vi "Encoder Position & Velocity (FPGA).vi"(3 "Velocity Interval (uSec)":u32=1000, 5 "Position Reset":bool) -> (0 "Right Velocity (Counts/Interval)":i32, 1 "Right Acceleration (Counts/Interval)":i32, 2 "Right Position (Counts)":i32)   [LabVIEW 2009]
doc: "This is an FPGA vi for Quadrature Encoder Velocity and Acceleration Estimation using CompactRIO. It requires as inputs a Fixed Time Interval for velocity and acceleration estimation.\n\nThis application is designed to work with an R-Series expansion setup using PCI/PXI-7811R FPGA device and a CompactRIO cRIO-9411 digital input module installed in slot 1 of the expansion chassis."
uses:
  <vilib>/rvi/Arithmetic/AddSubMult/XNode/nirviSatArithmetic.xnode
  <vilib>/eio/EIONode/EIONode.xnode
  <vilib>/rvi/eio/nirviEIOImplementation/nirviEIOImplementation.xnode
  <vilib>/rvi/eio/common/nirviEmuTemplateMethod_noerrors.vi
  <vilib>/rvi/eio/common/nirviEmuClasses.ctl
panel:
  in  "Velocity Interval (uSec) 2":u32=1000
  out "Left Position (Counts)":i32
  out "Left Acceleration (Counts/Interval)":i32
  out "Left Velocity (Counts/Interval)":i32
  in  "stop":bool
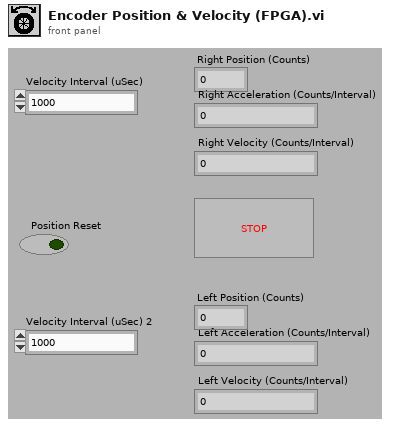
[diagram p1: front panel]
types:
  T1 = typedef "nirviEmuClasses.ctl" = enum16{"IO Read", "IO Write", "Method", "Property Read", "Property Write"}
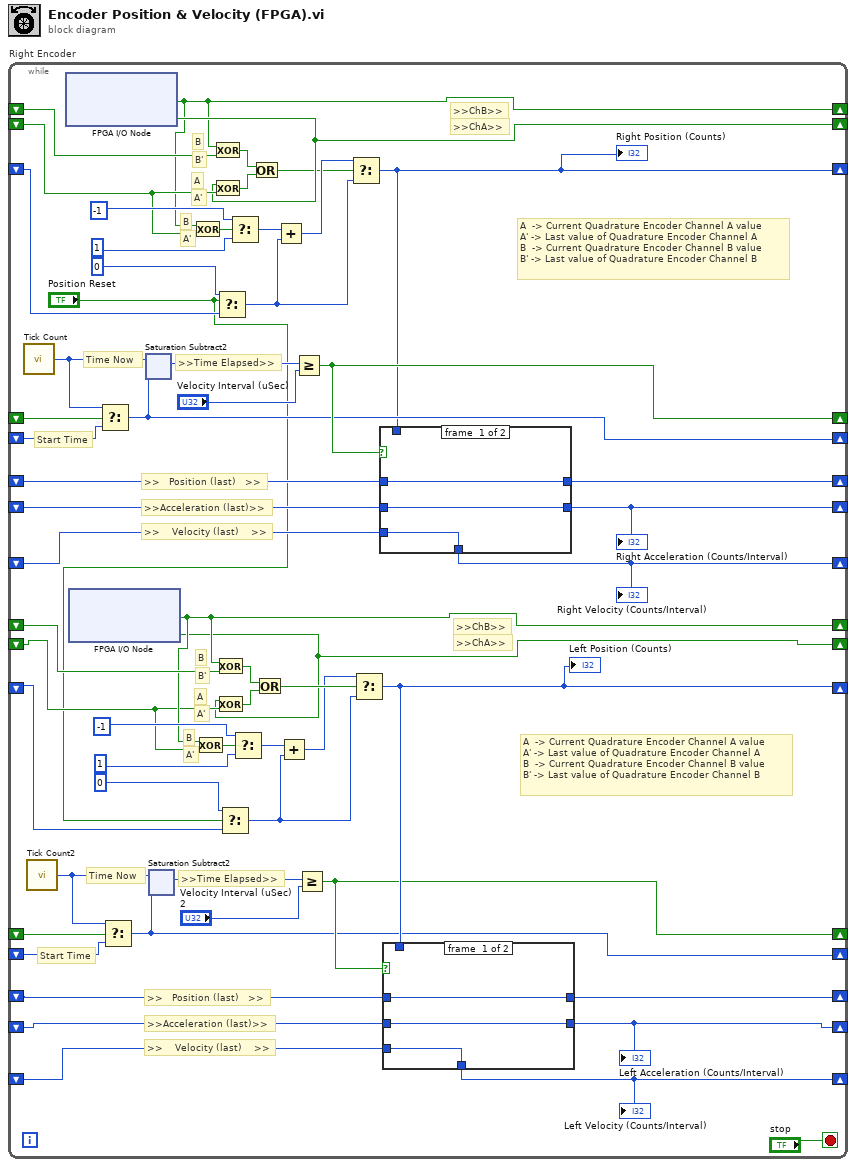
[diagram p0: block diagram]
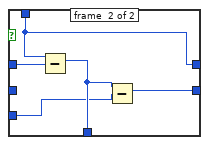
[diagram p2: hidden frame]
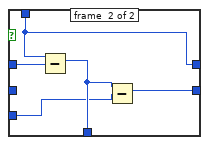
[diagram p3: hidden frame]
diagram:
  n1 = while "Right Encoder" {
    shift-right: [w32] -> _
    shift-left: _ -> [w36]
    shift-right: [w31] -> _
    shift-left: _ -> [w47]
    shift-right: [w50] -> _
    shift-left: _ -> [w51]
    shift-right: [w43] -> _
    shift-left: _ -> [w46]
    shift-right: [w38] -> _
    shift-left: _ -> [w44]
    shift-right: [w33] -> _
    shift-left: _ -> [w41]
    shift-right: [w34] -> _
    shift-left: _ -> [w40]
    shift-right: [w35] -> _
    shift-left: _ -> [w37]
    shift-right: [w16] -> _
    shift-left: _ -> [w17]
    shift-right: [w2] -> _
    shift-left: _ -> [w15]
    shift-right: [w13] -> _
    shift-left: _ -> [w14]
    shift-right: [w11] -> _
    shift-left: _ -> [w12]
    shift-right: [w9] -> _
    shift-left: _ -> [w10]
    shift-right: [w7] -> _
    shift-left: _ -> [w8]
    shift-right: [w4] -> _
    shift-left: _ -> [w6]
    shift-right: [w3] -> _
    shift-left: _ -> [w5]
    stop <- "stop" stop-if-true
    # "A  -> Current Quadrature Encoder Channel A value\nA' -> Last value of Quadrature Encoder Channel A\nB  -> Current Quadrature Encoder Channel B value\nB' -> Last value of Quadrature Encoder Channel B"
    # ">>Acceleration (last)>>"
    # "Start Time"
    # "A'"
    # "B"
    # "A'"
    # "A"
    # "B'"
    # "B"
    # ">>ChB>>"
    # ">>ChA>>"
    # ">>    Velocity (last)    >>"
    # ">>   Position (last)   >>"
    # "Time Now"
    # ">>Time Elapsed>>"
    # "A  -> Current Quadrature Encoder Channel A value\nA' -> Last value of Quadrature Encoder Channel A\nB  -> Current Quadrature Encoder Channel B value\nB' -> Last value of Quadrature Encoder Channel B"
    # ">>Acceleration (last)>>"
    # "Start Time"
    # "A'"
    # "B"
    # "A'"
    # "A"
    # "B'"
    # "B"
    # ">>ChB>>"
    # ">>ChA>>"
    # ">>    Velocity (last)    >>"
    # ">>   Position (last)   >>"
    # "Time Now"
    # ">>Time Elapsed>>"
    n2 = call "Tick Count"() -> ("Tick Count(uSec)"=w39:u32)
    n3 = call "Tick Count2"() -> ("Tick Count(uSec)"=w30:u32)
    n4 = xnode "FPGA I/O Node"() -> ("Mod2/DIO10"=w32:bool, "Mod2/DIO9"=w50:bool)  [unwired: 2 in, 2 out]
    n5 = xnode "FPGA I/O Node"() -> ("Mod2/DIO11"=w16:bool, "Mod2/DIO12"=w2:bool)  [unwired: 2 in, 2 out]
    n6 = Select(t=w39, s=w46, f=w44) -> (s? t:f=w38:u32)
    n7 = Select(t=w30, s=w12, f=w10) -> (s? t:f=w9:u32)
    n8 = xnode ("Saturation Subtract2")("x"=w39, "y"=w38) -> ("x-y"=w42:u32)
    n9 = xnode ("Saturation Subtract2")("x"=w30, "y"=w9) -> ("x-y"=w29:u32)
    n10 = Exclusive Or(1:w51, 2:w32) -> (0:w52:bool)
    n11 = Exclusive Or(1:w15, 2:w16) -> (0:w26:bool)
    n12 = Exclusive Or(1:w36, 2:w32) -> (0:w53:bool)
    n13 = Exclusive Or(1:w51, 2:w50) -> (0:w54:bool)
    n14 = Exclusive Or(1:w17, 2:w16) -> (0:w25:bool)
    n15 = Exclusive Or(1:w15, 2:w2) -> (0:w24:bool)
    n16 = Select(t=0 ("32 bit"), s="Position Reset", f=w47) -> (s? t:f=w58:i32)
    n17 = Select(t=0 ("32 bit"), s="Position Reset", f=w14) -> (s? t:f=w20:i32)
    n18 = Select(t=-1 ("32 bit"), s=w52, f=1 ("32 bit")) -> (s? t:f=w57:i32)
    n19 = Select(t=-1 ("32 bit"), s=w26, f=1 ("32 bit")) -> (s? t:f=w21:i32)
    n20 = Or(x=w53, y=w54) -> (x .or. y?=w48:bool)
    n21 = Or(x=w25, y=w24) -> (x .or. y?=w27:bool)
    n22 = Add(x=w57, y=w58) -> (x+y=w60:i32)
    n23 = Add(x=w21, y=w20) -> (x+y=w18:i32)
    n24 = Greater Or Equal?(x=w42, y="Velocity Interval (uSec)") -> (x >= y?=w43:bool)
    n25 = Greater Or Equal?(x=w29, y="Velocity Interval (uSec) 2") -> (x >= y?=w11:bool)
    n26 = Select(t=w60, s=w48, f=w58) -> (s? t:f=w31:i32)
    "Right Position (Counts)" <- w31
    n27 = Select(t=w18, s=w27, f=w20) -> (s? t:f=w13:i32)
    "Left Position (Counts)" <- w13
    n28 = case shown="True" w43 {
      tunnel: w31 -> [_ w168]
      tunnel: w41 -> [w165 w172]
      tunnel: [w167 w171] -> w34
      tunnel: w40 -> [w167 w170]
      tunnel: [w166 w169] -> w35
      tunnel: w37 -> [w166 _]
      tunnel: [w165 w168] -> w33
      frame #0 {
      }
      frame #1 {
        n29 = Subtract(x=w168, y=w172) -> (x-y=w171:i32)
        n30 = Subtract(x=w171, y=w170) -> (x-y=w169:i32)
      }
    }
    "Right Acceleration (Counts/Interval)" <- w35
    "Right Velocity (Counts/Interval)" <- w34
    n31 = case shown="True" w11 {
      tunnel: w13 -> [_ w112]
      tunnel: w8 -> [w109 w116]
      tunnel: [w111 w115] -> w3
      tunnel: w5 -> [w111 w114]
      tunnel: [w110 w113] -> w4
      tunnel: w6 -> [w110 _]
      tunnel: [w109 w112] -> w7
      frame #0 {
      }
      frame #1 {
        n32 = Subtract(x=w112, y=w116) -> (x-y=w115:i32)
        n33 = Subtract(x=w115, y=w114) -> (x-y=w113:i32)
      }
    }
    "Left Acceleration (Counts/Interval)" <- w4
    "Left Velocity (Counts/Interval)" <- w3
  }
